vi "Motor-Zera-Pos.vi"(2 "error":errorcluster, 3 "MG17Motor A":refnum<k7>) -> (0 "error out":errorcluster, 1 "MG17Motor out":refnum<k7>)   [LabVIEW 2014]
doc: "André Romero - 2016\nandretec@ifsc.usp.br\nIFSC - USP"
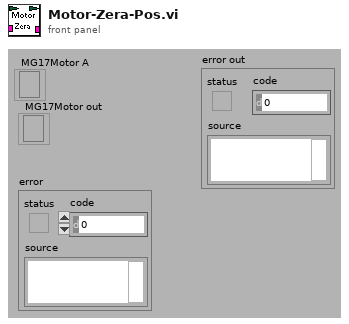
[diagram p1: front panel]
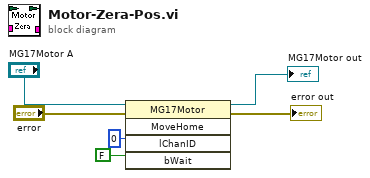
[diagram p0: block diagram]
diagram:
  n1 = invoke class="MG17Motor" method="MoveHome"(reference="MG17Motor A", error in="error", "lChanID"=0, "bWait"=FALSE) -> (reference out=→"MG17Motor out":refnum<k7>, error out=→"error out":errorcluster)  [unwired: 1 in, 3 out]
